vi "CRYSerial No Editor.vi"() -> ()   [LabVIEW 2013]
uses:
  <vilib>/Utility/miscctls.llb/LVBoundsTypeDef.ctl
  Typedef Control/CRYSerial No.ctl
  CRYProject/CRYProject Editor Global.vi
  CRYWindow/SubVI/CRYMain Sub Window Global.vi
  CRYMainGlobal.vi
panel:
  out "Serial# Bk":T1
  out "EndFlag":bool
  in  "AddStep":bool
  out "Serial#":T1
  in  "Load Test":bool caption="Load"
  out "VIMiniumBound":T2
  out "Proper VI No":i32
  in  "Board Tab":enum32{"Page 1", "Page 2"}(tab)
  in  "Cancel":bool caption="Apply"
  in  "OK":bool caption="Apply"
  in  "Main Tab":enum32{"Setting", "Help"}(tab)
  in  "S/N Prefix":string="0" caption="S/N前缀"
  in  "Mode":u16(slide)=1
  out "Selection":bool caption="选择"
  in  "Help":string
  in  "Load...":bool caption="Apply"
  in  "Revert":bool caption="Apply"
  in  "Save As...":bool caption="Apply"
  in  "stop":bool
  in  "Channel":i32=1
  in  "Hardware in":string
  in  "Calibration in":string
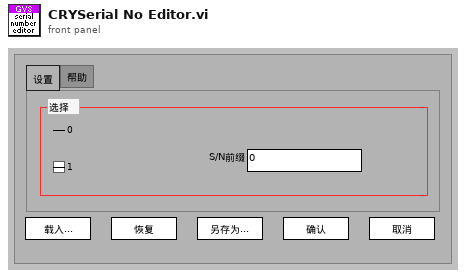
[diagram p1: front panel]
types:
  T1 = typedef "CRYSerial No.ctl" = cluster{"Name":string, "Mode":u16, "S/N prefix":string, "Tab Value":u16, "Help":string}
  T2 = typedef "LVBoundsTypeDef.ctl" = cluster{"Width":u32, "Height":u32}
  T3 = typedef "CRYStep.ctl" = cluster{"No.VI":i32, "Category":string, "StepName":string, "Seq setup flattened":string, "Comment":string, "Steps config.":bool[], "Jump config":i32[], "Start":dbl, "Increment":dbl, "Name":string, "Unit":string, "Y data":u16, "Y prefix":string, "Y dB ref":dbl, "Y unit":string, "Repeat State Array":cluster{"Start":dbl, "Increment":dbl, "Count":i32, "Num":i32}[]}
  T4 = enum16{"OK", "Yes", "YesNo", "YesNoCancel", "ReplaceAppend"}
  T5 = enum8{"Enabled", "Disabled", "Disabled and Grayed Out"}
  T6 = cluster{"Load Test":bool, "OK":bool, "Cancel":bool}
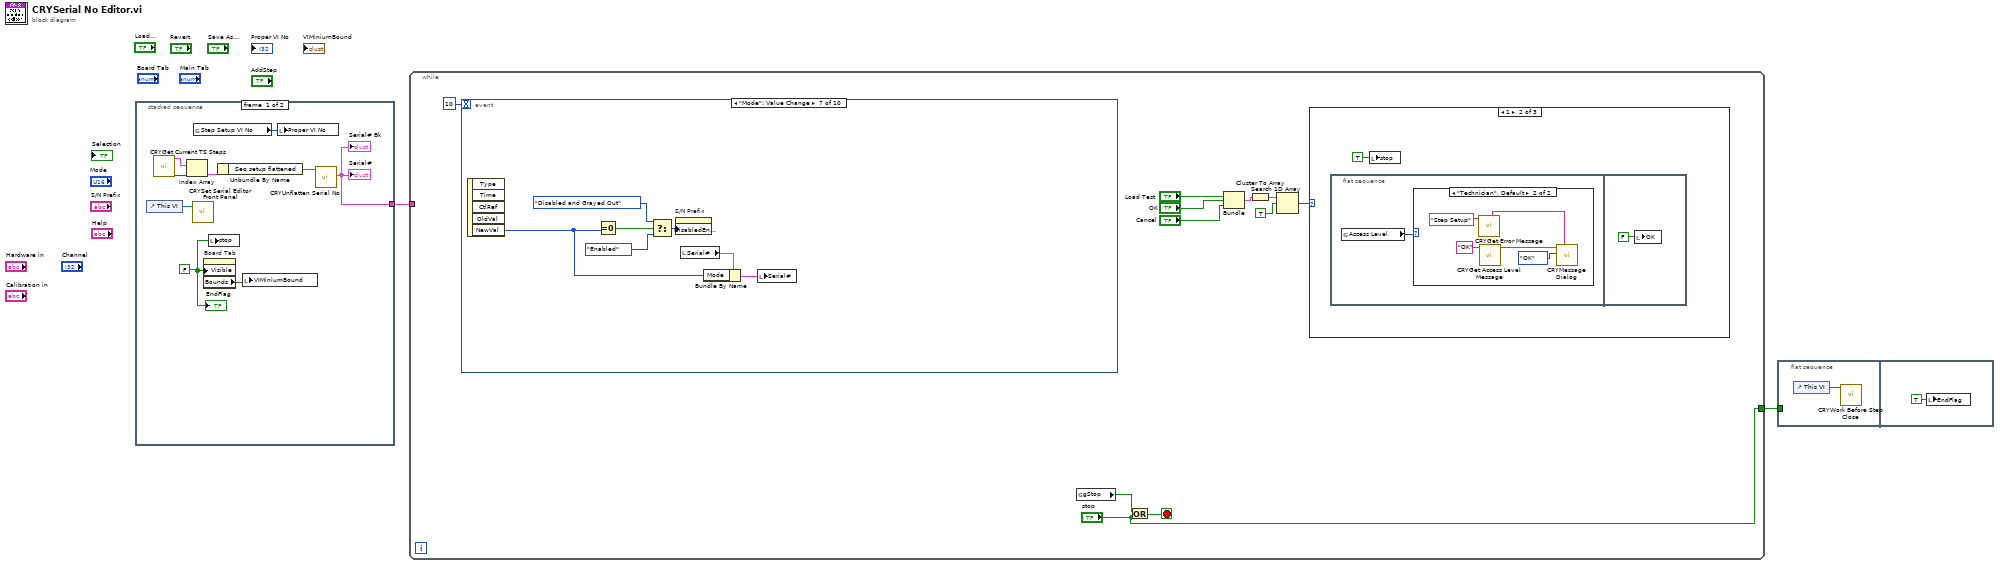
[diagram p0: block diagram]
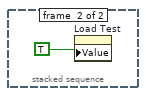
[diagram p2: hidden frame]
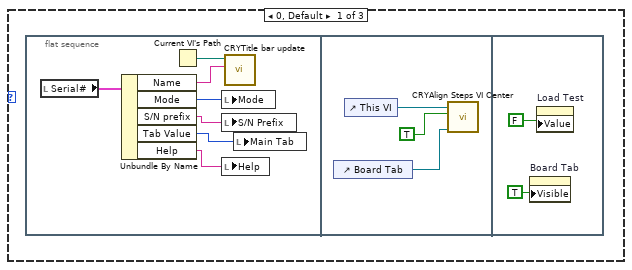
[diagram p3: hidden frame]
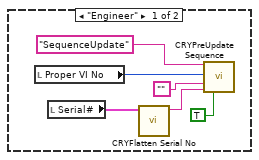
[diagram p4: hidden frame]
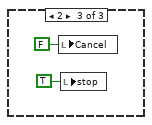
[diagram p5: hidden frame]
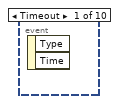
[diagram p6: hidden frame]
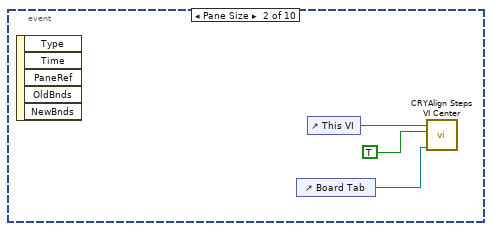
[diagram p7: hidden frame]
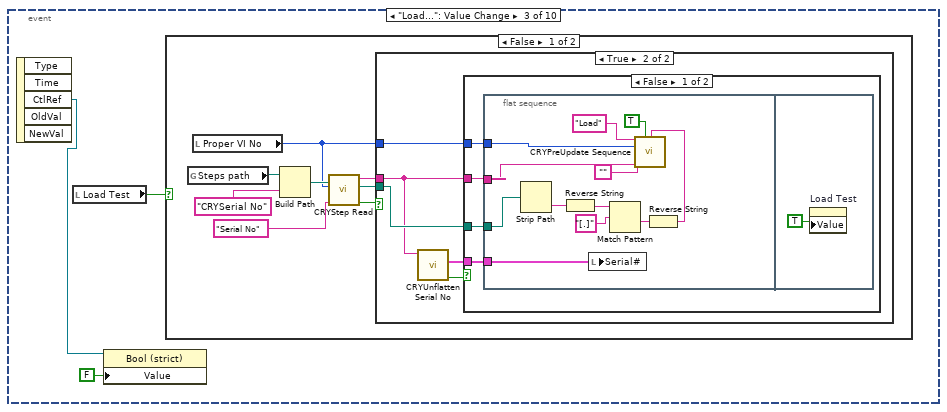
[diagram p8: hidden frame]
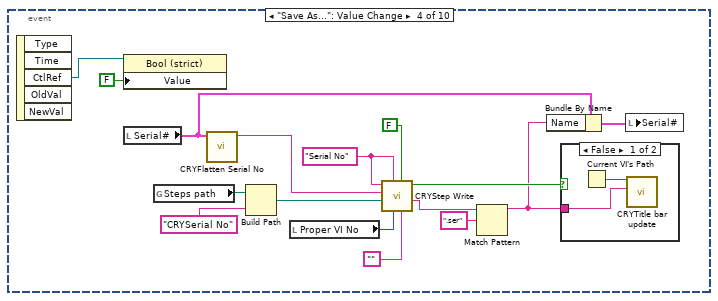
[diagram p12: hidden frame]
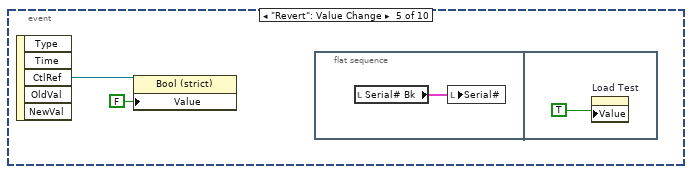
[diagram p14: hidden frame]
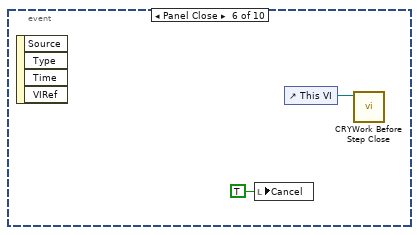
[diagram p15: hidden frame]
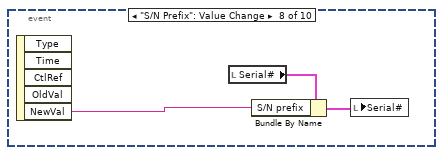
[diagram p16: hidden frame]
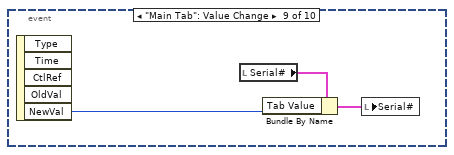
[diagram p17: hidden frame]
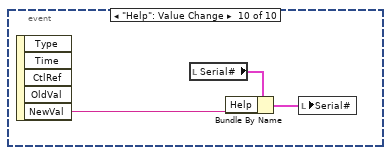
[diagram p18: hidden frame]
diagram:
  n1 = stacked-sequence {
    tunnel: [w4 _] -> w2
    frame #0 {
      w3 = FALSE ("Visible")
      n2 = control-ref of="This VI"() -> (w5:refnum<vi>)
      n3 = call "CRYGet Current TS Steps.vi"() -> ("SelectStepNumber in Tree"=w9:i32, "Steps"=w10:T3[])  [unwired: 7 in, 3 out]
      n4 = Index Array(array=w10, index=w9) -> (element=w11:T3)
      n5 = call "CRYSet Serial Editor Front Panel.vi"("Vi Ref"=w5) -> ()  [unwired: 11 in]
      n6 = global read "CRYProject Editor Global.vi" "Step Setup VI No"() -> (w8:i32)
      n7 = property on="Board Tab" class="TabCtl (strict)"("Visible"=w3) -> ("Bounds"=w7:T2)  [unwired: 2 in, 2 out]
      n8 = local write "stop"(w3) -> ()
      n9 = Unbundle By Name(w11) -> ("Seq setup flattened"=w6:string)
      n10 = local write "VIMiniumBound"(w7) -> ()
      n11 = local write "Proper VI No"(w8) -> ()
      n12 = call "CRYUnflatten Serial No.vi"("Unflatten Serial#"=w6) -> ("Serial#"=w4:T1)  [unwired: 8 in, 2 out]
      "Serial#" <- w4
      "Serial# Bk" <- w4
      "EndFlag" <- w3
    }
    frame #1 {
      n13 = property on="Load Test" class="Bool (strict)"("Value"=TRUE ("Load Test")) -> ()  [unwired: 2 in, 2 out]
    }
  }
  n14 = while {
    tunnel: w2 -> [_]
    tunnel: ["stop"] -> w1
    stop <- w21 stop-if-true
    n15 = event shown="[6] \"Mode\": Value Change" {
      selector: _ -> [_ _ _ _ _ _ _ _ _ _]
      dyn-events: _ -> [_ _ _ _ _ _ _ _ _ _]
      timeout: 10 -> [_ _ _ _ _ _ _ _ _ _]
      event Timeout {
        n16 = event-data() -> ()  [unwired: 1 in, 2 out]
      }
      event Pane Size {
        n17 = event-data() -> ()  [unwired: 1 in, 5 out]
        n18 = control-ref of="Board Tab"() -> (w52:refnum<vi>)
        n19 = control-ref of="This VI"() -> (w54:refnum<vi>)
        n20 = call "CRYAlign Steps VI Center.vi"("Tab2"=w52, "Input/Output"=TRUE, "VIRef"=w54) -> ()  [unwired: 1 in, 8 out]
      }
      event "Load...": Value Change {
        n21 = event-data() -> ("CtlRef"=w55:refnum<vi>)  [unwired: 1 in, 4 out]
        n22 = local read "Load Test"() -> (w57:bool)
        n23 = property class="Bool (strict)"(reference=w55, "Value"=FALSE) -> ()  [unwired: 1 in, 2 out]
        n24 = case shown="False" w57 {
          frame False {
            n25 = global read "CRYMainGlobal.vi" "Steps path"() -> (w64:path)
            n26 = local read "Proper VI No"() -> (w58:i32)
            n27 = Build Path(base path=w64, name or relative path="CRYSerial No") -> (appended path=w65:path)
            n28 = call "CRYStep Read.vi"("Category Name"="Serial No" ("Step File Name"), "Proper VI No"=w58, "Step File Path"=w65) -> ("status"=w61:bool, "selected path"=w59:path, "Flatten Step"=w60:string)  [unwired: 1 in, 3 out]
            n29 = case shown="True" w61 {
              tunnel: w60 -> [_ w67]
              tunnel: w59 -> [_ w68]
              tunnel: w58 -> [_ w66]
              frame False {
              }
              frame True {
                n30 = call "CRYUnflatten Serial No.vi"("Unflatten Serial#"=w67) -> ("Error?"=w70:bool, "Serial#"=w69:T1)  [unwired: 8 in, 1 out]
                n31 = case shown="False" w70 {
                  tunnel: w69 -> [w74 _]
                  tunnel: w68 -> [w73 _]
                  tunnel: w67 -> [w72 _]
                  tunnel: w66 -> [w71 _]
                  frame False {
                    n32 = flat-sequence {
                      tunnel: w74 -> [w86]
                      tunnel: w73 -> [w83]
                      tunnel: w72 -> [w82]
                      tunnel: w71 -> [w81]
                      frame #0 {
                        n33 = Strip Path(path=w83) -> (name=w76:string)  [unwired: 1 out]
                        n34 = Reverse String(1:w76) -> (0:w78:string)
                        n35 = local write "Serial#"(w86) -> ()
                        n36 = Match Pattern(string=w78, regular expression="[.]") -> (after substring=w79:string)  [unwired: 4 out]
                        n37 = Reverse String(1:w79) -> (0:w75:string)
                        n38 = call "CRYPreUpdate Sequence.vi"("EventName"="Load", "StepName Arg3"=w75, "Proper VI No"=w81, "Project View Step Name Identifier Arg1"="", "Step flattened Arg2"=w82, "AllChangeFlg"=TRUE ("Name/Identifier")) -> ()  [unwired: 10 in]
                      }
                      frame #1 {
                        n39 = property on="Load Test" class="Bool (strict)"("Value"=TRUE ("Load Test")) -> ()  [unwired: 2 in, 2 out]
                      }
                    }
                  }
                  frame True {
                  }
                }
              }
            }
          }
          frame True {
          }
        }
      }
      event "Save As...": Value Change {
        w97 = "Serial No" ("Step File Name")
        n40 = event-data() -> ("CtlRef"=w88:refnum<vi>)  [unwired: 1 in, 4 out]
        n41 = property class="Bool (strict)"(reference=w88, "Value"=FALSE) -> ()  [unwired: 1 in, 2 out]
        n42 = local read "Serial#"() -> (w92:T1)
        n43 = global read "CRYMainGlobal.vi" "Steps path"() -> (w103:path)
        n44 = call "CRYFlatten Serial No.vi"("Serial#"=w92) -> ("Serial# flattened"=w96:string)  [unwired: 10 in]
        n45 = Build Path(base path=w103, name or relative path="CRYSerial No") -> (appended path=w99:path)
        n46 = local read "Proper VI No"() -> (w98:i32)
        n47 = call "CRYStep Write.vi"("StepIdentifier"="", "Default"=FALSE, "Proper VI No"=w98, "Category Name"=w97, "Step File Path"=w99, "Step flattened"=w96, "Step File Name"=w97) -> ("name"=w94:string, "Cancel"=w95:bool)  [unwired: 1 in, 2 out]
        n48 = Match Pattern(string=w94, regular expression=".ser") -> (before substring=w91:string)  [unwired: 1 in, 3 out]
        n49 = Bundle By Name(cluster=w92, "Name"=w91) -> (w90:T1)
        n50 = case shown="False" w95 {
          tunnel: w91 -> [w104 _]
          frame False {
            n51 = Current VI's Path() -> (path=w105:path)
            n52 = call "CRYTitle bar update.vi"("Step name"=w104, "Editor VI path"=w105) -> ()  [unwired: 10 in]
          }
          frame True {
          }
        }
        n53 = local write "Serial#"(w90) -> ()
      }
      event "Revert": Value Change {
        n54 = event-data() -> ("CtlRef"=w106:refnum<vi>)  [unwired: 1 in, 4 out]
        n55 = property class="Bool (strict)"(reference=w106, "Value"=FALSE) -> ()  [unwired: 1 in, 2 out]
        n56 = flat-sequence {
          frame #0 {
            n57 = local read "Serial# Bk"() -> (w108:T1)
            n58 = local write "Serial#"(w108) -> ()
          }
          frame #1 {
            n59 = property on="Load Test" class="Bool (strict)"("Value"=TRUE ("Load Test")) -> ()  [unwired: 2 in, 2 out]
          }
        }
      }
      event Panel Close {
        n60 = event-data() -> ()  [unwired: 1 in, 4 out]
        n61 = local write "Cancel"(TRUE ("Cancel")) -> ()
        n62 = control-ref of="This VI"() -> (w111:refnum<vi>)
        n63 = call "CRYWork Before Step Close.vi"("StepVI Ref"=w111) -> ()  [unwired: 11 in]
      }
      event "Mode": Value Change {
        n64 = event-data() -> ("NewVal"=w113:u16)  [unwired: 1 in, 4 out]
        n65 = Equal To 0?(x=w113) -> (x = 0?=w118:bool)
        n66 = Select(t=T5."Disabled and Grayed Out", s=w118, f=T5."Enabled" ("Disabled")) -> (s? t:f=w115:T5)
        n67 = property on="S/N Prefix" class="Str"("DisabledEnum"=w115) -> ()  [unwired: 2 in, 2 out]
        n68 = local read "Serial#"() -> (w114:T1)
        n69 = Bundle By Name(cluster=w114, "Mode"=w113) -> (w112:T1)
        n70 = local write "Serial#"(w112) -> ()
      }
      event "S/N Prefix": Value Change {
        n71 = event-data() -> ("NewVal"=w120:string)  [unwired: 1 in, 4 out]
        n72 = local read "Serial#"() -> (w121:T1)
        n73 = Bundle By Name(cluster=w121, "S/N prefix"=w120) -> (w119:T1)
        n74 = local write "Serial#"(w119) -> ()
      }
      event "Main Tab": Value Change {
        n75 = event-data() -> ("NewVal"=w123:enum32{"Setting", "Help"})  [unwired: 1 in, 4 out]
        n76 = local read "Serial#"() -> (w124:T1)
        n77 = Bundle By Name(cluster=w124, "Tab Value"=w123) -> (w122:T1)
        n78 = local write "Serial#"(w122) -> ()
      }
      event "Help": Value Change {
        n79 = event-data() -> ("NewVal"=w126:string)  [unwired: 1 in, 4 out]
        n80 = local read "Serial#"() -> (w127:T1)
        n81 = Bundle By Name(cluster=w127, "Help"=w126) -> (w125:T1)
        n82 = local write "Serial#"(w125) -> ()
      }
    }
    n83 = global read "CRYMain Sub Window Global.vi" "gStop"() -> (w22:bool)
    n84 = Or(x=w22, y="stop") -> (x .or. y?=w21:bool)
    n85 = Bundle("Load Test"="Load Test", "OK"="OK", "Cancel"="Cancel") -> (w20:T6)  [unwired: 1 out]
    n86 = Cluster To Array(cluster=w20) -> (array=w19:bool[])
    n87 = Search 1D Array(1D array=w19, element=TRUE) -> (index of element=w16:i32)  [unwired: 1 out]
    n88 = case shown="1" w16 {
      frame 0, Default {
        n89 = flat-sequence {
          frame #0 {
            n90 = local read "Serial#"() -> (w30:T1)
            n91 = Unbundle By Name(w30) -> ("Name"=w24:string, "Mode"=w29:u16, "S/N prefix"=w28:string, "Tab Value"=w27:u16, "Help"=w26:string)
            n92 = Current VI's Path() -> (path=w25:path)
            n93 = local write "Mode"(w29) -> ()
            n94 = local write "S/N Prefix"(w28) -> ()
            n95 = local write "Help"(w26) -> ()
            n96 = call "CRYTitle bar update.vi"("Step name"=w24, "Editor VI path"=w25) -> ()  [unwired: 10 in]
            n97 = local write "Main Tab"(w27) -> ()
          }
          frame #1 {
            n98 = control-ref of="Board Tab"() -> (w31:refnum<vi>)
            n99 = control-ref of="This VI"() -> (w33:refnum<vi>)
            n100 = call "CRYAlign Steps VI Center.vi"("Tab2"=w31, "Input/Output"=TRUE, "VIRef"=w33) -> ()  [unwired: 1 in, 8 out]
          }
          frame #2 {
            n101 = property on="Board Tab" class="TabCtl (strict)"("Visible"=TRUE) -> ()  [unwired: 2 in, 2 out]
            n102 = property on="Load Test" class="Bool (strict)"("Value"=FALSE ("Load Test")) -> ()  [unwired: 2 in, 2 out]
          }
        }
      }
      frame 1 {
        n103 = flat-sequence {
          frame #0 {
            n104 = global read "CRYMainGlobal.vi" "Access Level"() -> (w37:enum16{"Engineer", "Technician", "Operator"})
            n105 = case shown="\"Technician\", Default" w37 {
              frame "Engineer" {
                n106 = local read "Proper VI No"() -> (w41:i32)
                n107 = local read "Serial#"() -> (w40:T1)
                n108 = call "CRYFlatten Serial No.vi"("Serial#"=w40) -> ("Serial# flattened"=w39:string)  [unwired: 10 in]
                n109 = call "CRYPreUpdate Sequence.vi"("EventName"="SequenceUpdate", "Proper VI No"=w41, "Project View Step Name Identifier Arg1"="", "Step flattened Arg2"=w39, "AllChangeFlg"=TRUE ("Name/Identifier")) -> ()  [unwired: 11 in]
              }
              frame "Technician", Default {
                n110 = call "CRYGet Error Message.vi"("Kind"="Step Setup") -> ("Window Title"=w46:string)  [unwired: 5 in, 5 out]
                n111 = call "CRYGet Access Level Message.vi"("sAction"="OK") -> ("Multibyte string"=w48:string)  [unwired: 10 in]
                n112 = call "CRYMessage Dialog.vi"("Window Title"=w46, "YesNoCancel"=T4."OK", "Message Content"=w48) -> ()  [unwired: 7 in, 2 out]
              }
            }
          }
          frame #1 {
            n113 = local write "OK"(FALSE ("OK")) -> ()
          }
        }
        n114 = local write "stop"(TRUE ("stop")) -> ()
      }
      frame 2 {
        n115 = local write "Cancel"(FALSE ("Cancel")) -> ()
        n116 = local write "stop"(TRUE ("stop")) -> ()
      }
    }
  }
  n117 = flat-sequence {
    tunnel: w1 -> [_]
    frame #0 {
      n118 = control-ref of="This VI"() -> (w128:refnum<vi>)
      n119 = call "CRYWork Before Step Close.vi"("StepVI Ref"=w128) -> ()  [unwired: 11 in]
    }
    frame #1 {
      n120 = local write "EndFlag"(TRUE ("EndFlag")) -> ()
    }
  }
